vi "Get IConfiguration.vi"(11 "IConfigure in":refnum<class "IConfigure.lvclass">) -> (2 "IConfiguration":refnum<class "IConfiguration.lvclass">, 3 "IConfigure out":refnum<class "IConfigure.lvclass">)   [LabVIEW 2019, in "IConfigure.lvclass"]
uses:
  IConfigure.lvclass
  IConfiguration/IConfiguration.lvclass
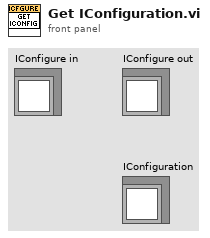
[diagram p1: front panel]
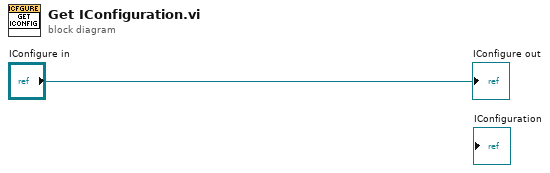
[diagram p0: block diagram]
diagram:
  "IConfigure out" <- "IConfigure in"
